vi "loadHTSocketContactYield.vi"(11 "file (use dialog)":path=path "C:/temp/ht/Socket/MSD6A638JSMG-8-Y8_A151200729_EQC_151220030900.txt") -> ()   [LabVIEW 2012]
uses:
  <vilib>/addons/database/Connection.llb/DB Tools Open Connec (Path).vi
  <vilib>/addons/database/Connection.llb/Conn Execute.vi
  <vilib>/addons/database/Recordset.llb/Rec Destroy - Connection.vi
  <vilib>/addons/database/NI_Database_API.lvlib
panel:
  out "array":string[][](array[string])
  out "concatenated string":string
  out "error out":errorcluster
  out "name":string
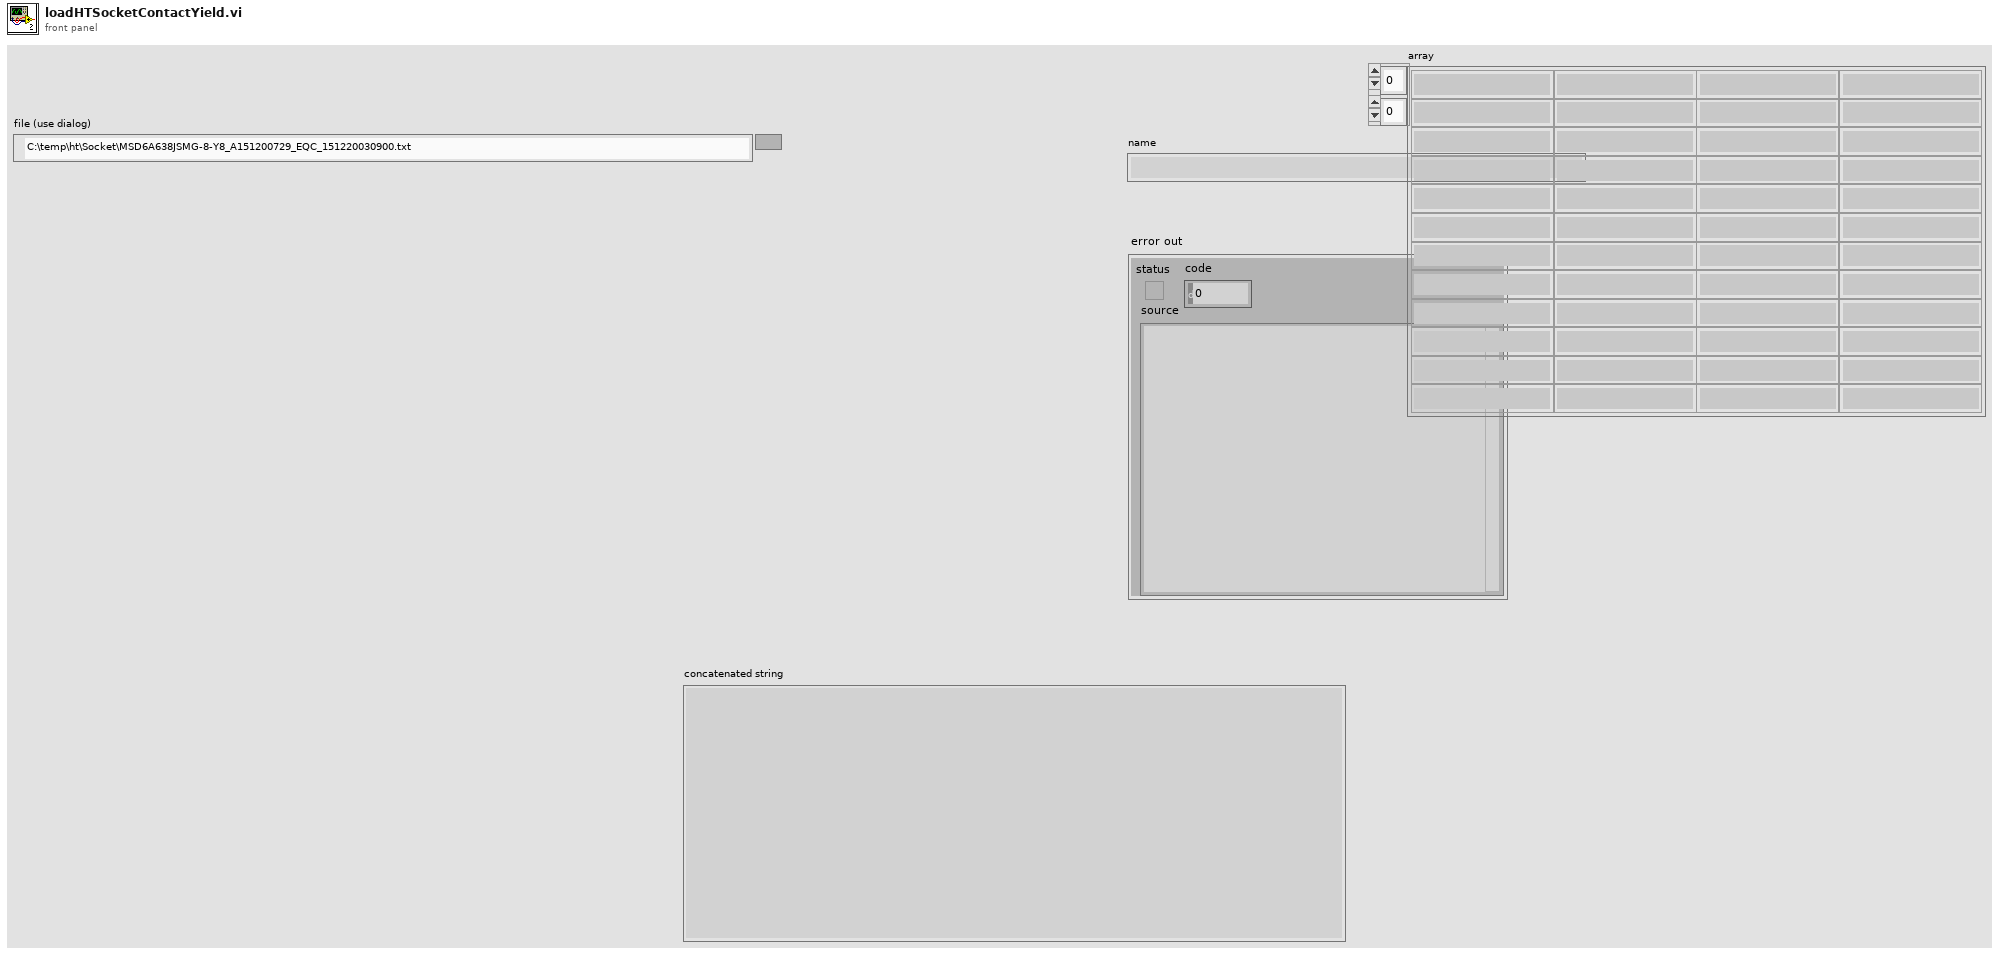
[diagram p1: front panel]
types:
  T1 = typedef "NI_Database_API.lvlib/Conn ObjectReference.ctl" = refnum<k1>
  T2 = typedef "NI_Database_API.lvlib/Rec ObjectReference.ctl" = refnum<k1>
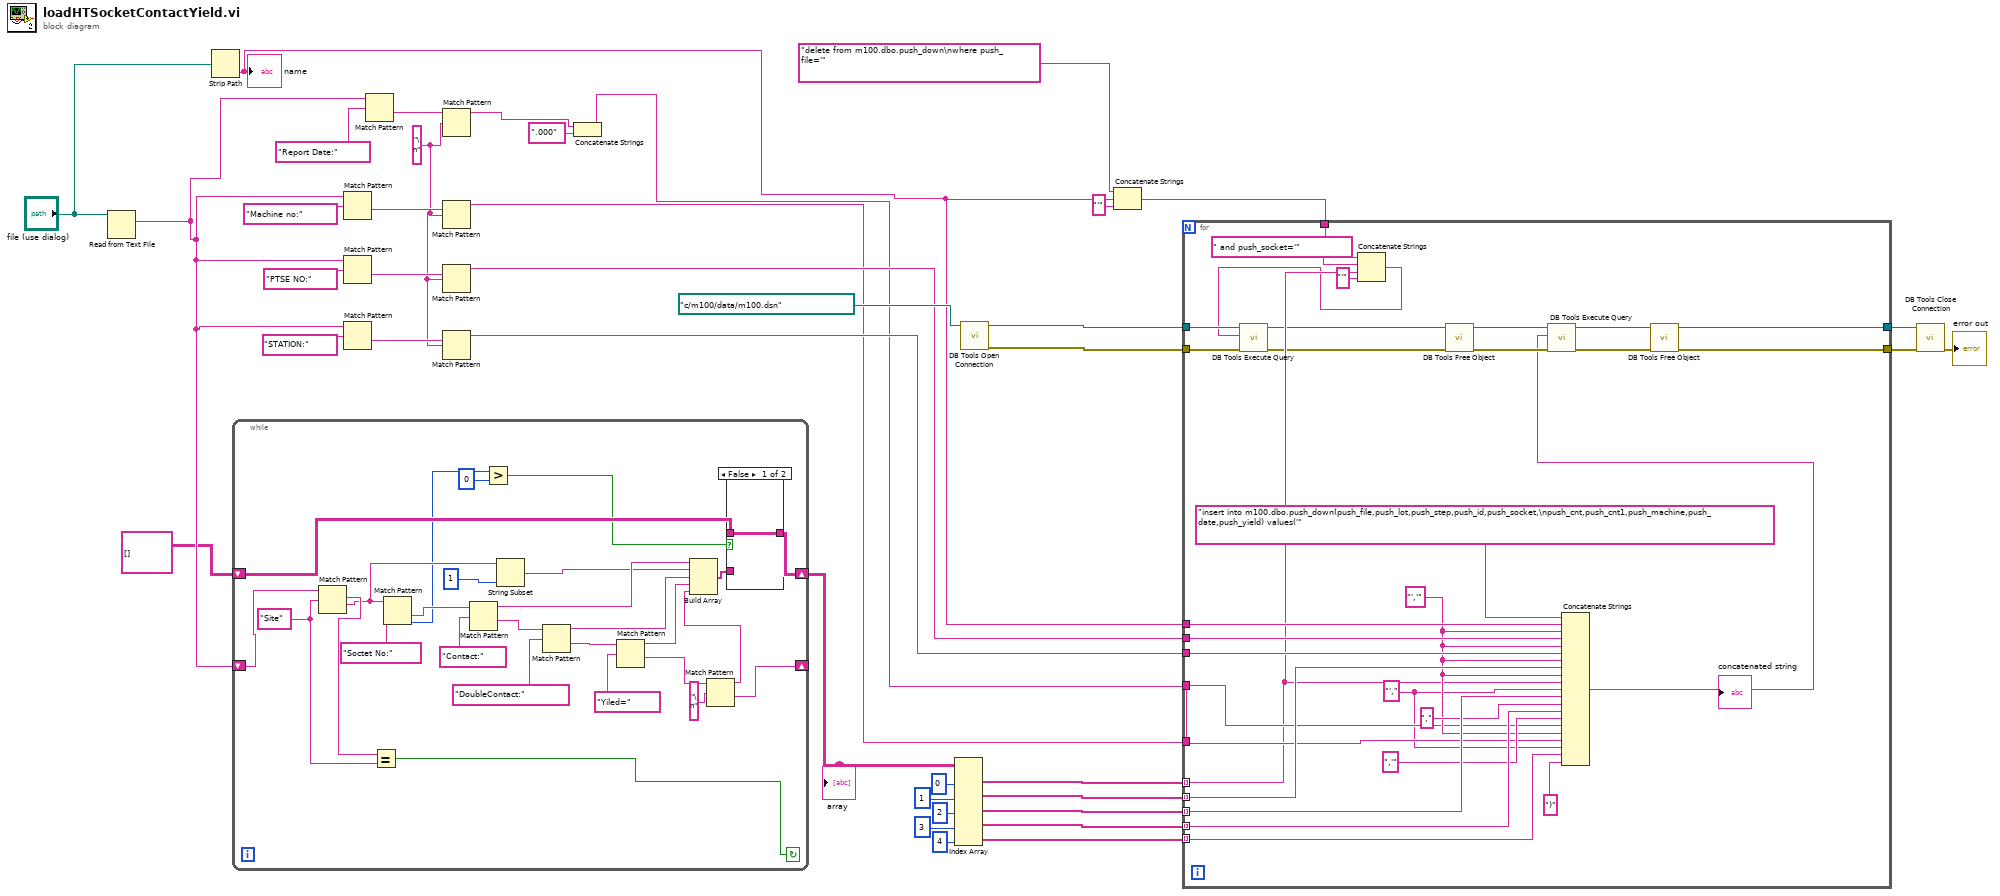
[diagram p0: block diagram]
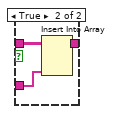
[diagram p2: hidden frame]
diagram:
  w28 = "\n" ("regular expression")
  n1 = Read from Text File(file (use dialog)="file (use dialog)") -> (text=w5:string)  [unwired: 3 in, 3 out]
  n2 = Strip Path(path="file (use dialog)") -> (name=w18:string)  [unwired: 1 out]
  "name" <- w18
  n3 = while {
    shift-right: [w42] -> _
    shift-left: w5 -> [w55]
    shift-right: [w54] -> w3
    shift-left: string[][] [] ("array") -> [w53]
    stop <- w50 continue-if-true
    w51 = "Site" ("regular expression")
    n4 = Match Pattern(string=w55, regular expression=w51) -> (match substring=w52:string, after substring=w47:string)  [unwired: 1 in, 2 out]
    n5 = Equal?(x=w52, y=w51) -> (x = y?=w50:bool)
    n6 = Match Pattern(string=w47, regular expression="Soctet No:") -> (after substring=w49:string, offset past match=w46:i32)  [unwired: 1 in, 2 out]
    n7 = Match Pattern(string=w49, regular expression="Contact:") -> (before substring=w65:string, after substring=w63:string)  [unwired: 1 in, 2 out]
    n8 = Greater?(x=w46, y=0) -> (0:w44:bool)
    n9 = String Subset(string=w47, length (rest)=1 ("length (rest)")) -> (substring=w56:string)  [unwired: 1 in]
    n10 = Match Pattern(string=w63, regular expression="DoubleContact:") -> (before substring=w59:string, after substring=w61:string)  [unwired: 1 in, 2 out]
    n11 = Match Pattern(string=w61, regular expression="Yiled=") -> (before substring=w58:string, after substring=w43:string)  [unwired: 1 in, 2 out]
    n12 = Match Pattern(string=w43, regular expression="\n") -> (before substring=w40:string, after substring=w42:string)  [unwired: 1 in, 2 out]
    n13 = Build Array(w65, w56, w59, w58, w40) -> (w64:string[])
    n14 = case shown="False" w44 {
      tunnel: w64 -> [_ w70]
      tunnel: [w67 w69] -> w54
      tunnel: w53 -> [w67 w68]
      frame False {
      }
      frame True {
        n15 = Insert Into Array(array=w68, new element=w70) -> (w69:string[][])  [unwired: 2 in]
      }
    }
  }
  "array" <- w3
  n16 = Match Pattern(string=w5, regular expression="Machine no:") -> (after substring=w38:string)  [unwired: 1 in, 3 out]
  n17 = Match Pattern(string=w5, regular expression="PTSE NO:") -> (after substring=w31:string)  [unwired: 1 in, 3 out]
  n18 = Match Pattern(string=w5, regular expression="STATION:") -> (after substring=w29:string)  [unwired: 1 in, 3 out]
  n19 = Match Pattern(string=w5, regular expression="Report Date:") -> (after substring=w33:string)  [unwired: 1 in, 3 out]
  n20 = Match Pattern(string=w33, regular expression=w28) -> (before substring=w9:string)  [unwired: 1 in, 3 out]
  n21 = Match Pattern(string=w38, regular expression=w28) -> (before substring=w6:string)  [unwired: 1 in, 3 out]
  n22 = Match Pattern(string=w31, regular expression=w28) -> (before substring=w17:string)  [unwired: 1 in, 3 out]
  n23 = Match Pattern(string=w29, regular expression=w28) -> (before substring=w16:string)  [unwired: 1 in, 3 out]
  n24 = Concatenate Strings(w9, ".000" ("string")) -> (w7:string)
  n25 = Index Array(array=w3, index (col) #1=0 ("disabled index (col)"), index (col) #2=1 ("index (col)"), index (col) #3=2 ("index (col)"), index (col) #4=3 ("index (col)"), index (col) #5=4 ("index (col)")) -> (element #1=w12:string[], element #2=w13:string[], element #3=w11:string[], element #4=w10:string[], element #5=w1:string[])  [unwired: 5 in]
  n26 = call-poly <vilib>:"DB Tools Open Connection.vi"("connection information"=path "c:/m100/data/m100.dsn") -> ("error out"=w25:errorcluster, "connection reference"=w27:T1)  [unwired: 7 in]
  n27 = Concatenate Strings("delete from m100.dbo.push_down\nwhere push_file='", w18, "'" ("string")) -> (w19:string)
  n28 = for {
    tunnel: w27 -> [w101]
    tunnel: [w99] -> w26
    tunnel: w25 -> [w98]
    tunnel: [w96] -> w24
    tunnel: w19 -> [w82]
    tunnel: w18 -> [w94]
    tunnel: w17 -> [w93]
    tunnel: w16 -> [w92]
    tunnel: w13 -> [w91] mode=indexing
    tunnel: w12 -> [w80] mode=indexing
    tunnel: w11 -> [w90] mode=indexing
    tunnel: w10 -> [w88] mode=indexing
    tunnel: w7 -> [w85]
    tunnel: w6 -> [w83]
    tunnel: w1 -> [w76] mode=indexing
    w75 = "'," ("string")
    w84 = "','" ("string")
    n29 = Concatenate Strings(w82, " and push_socket='" ("string"), w80, "'" ("string")) -> (w78:string)
    n30 = call-poly <vilib>:"DB Tools Execute Query.vi"("error in (no error)"=w98, "SQL query"=w78, "connection reference"=w101) -> ("error out"=w71:errorcluster, "recordset reference"=w72:T2)  [unwired: 5 in]
    n31 = call-poly <vilib>:"DB Tools Free Object.vi"("error in (no error)"=w71, "recordset reference"=w72) -> ("error out"=w97:errorcluster, "connection reference"=w100:T1)  [unwired: 8 in]
    n32 = Concatenate Strings("insert into m100.dbo.push_down(push_file,push_lot,push_step,push_id,push_socket,\npush_cnt,push_cnt1,push_machine,push_date,push_yield) values('", w94, w84, w93, w84, w92, w84, w91, w84, w80, w75, w90, "," ("string"), w88, ",'" ("string"), w83, w84, w85, w75, w76, ")" ("string")) -> (w86:string)
    "concatenated string" <- w86
    n33 = call-poly <vilib>:"DB Tools Execute Query.vi"("error in (no error)"=w97, "SQL query"=w86, "connection reference"=w100) -> ("error out"=w73:errorcluster, "recordset reference"=w74:T2)  [unwired: 5 in]
    n34 = call-poly <vilib>:"DB Tools Free Object.vi"("error in (no error)"=w73, "recordset reference"=w74) -> ("error out"=w96:errorcluster, "connection reference"=w99:T1)  [unwired: 8 in]
  }
  n35 = call <vilib>:"DB Tools Close Connection.vi"("error in (no error)"=w24, "connection reference"=w26) -> ("error out"=→"error out":errorcluster)  [unwired: 5 in]
